vi "Convert_Always_Show_Info.vi"(0 "Array":T9[](array[typedef]) {"ERD Number" format="%.0x"}, 1 "Version":T7, 2 "ATC Data":T3, 5 "Raw Data Out":string[](array[string]), 7 "Previous ERD Info":T8, 9 "ERD Graph Cntrl":T4 {"ERD 1"."Scaler" min=1; "ERD 1"."ERD #" format="%.0x"; "ERD 2"."Scaler" min=1; "ERD 2"."ERD #" format="%.0x"; "ERD 3"."Scaler" min=1; "ERD 3"."ERD #" format="%.0x"}, 11 "Error In":errorcluster) -> (3 "Version":T7, 4 "ERD_Always Show":T8, 6 "Redundant Micro":T6, 8 "ATC Data":T3, 10 "ERD Graph  Ind":T1, 13 "Numeric":i32, 14 "Algorithm Data 2":T2, 15 "Error Out":errorcluster)   [LabVIEW 2014]
doc: "This VI parses the data from ERDs in correct format, units, etc. It handles all hex to dec conversions, hex to enum, and hex to boolean conversions.\n\nIf Raw Data from ERD is blank string, then it will output values from shift register."
uses:
  Utility/LabVIEW GEA2 Toolkit v1.0.0.0/type defs/ERD Read Data Out.ctl
  Utility/LabVIEW GEA2 Toolkit v1.0.0.0/library/GEA2_Toolkit.lvlib
  type defs/ERD_Always_Show.ctl
  type defs/Version.ctl
  type defs/Redundant.ctl
  type defs/ERD_Graph.ctl
  type defs/ERD_Graph_All.ctl
  type defs/ATC_Data.ctl
  type defs/Algorithms.ctl
panel:
  in  "ERD Graph  Ind":T1
  in  "Algorithm Data":T2
  in  "Redundant Micro":T6
  # "Wet Load Size"
  # "Dry Load Size"
  # "OOB"
  # "Wet Load Size"
  # "Dry Load Size"
  # "OOB"
  # "Software Version"
  # "Critical Version"
  # "Non-Critical"
  # "XML Crit Ver"
  # "XML Non-Crit"
  # "Daily Build"
  # "Software Version"
  # "Critical Version"
  # "Non-Critical"
  # "XML Crit Ver"
  # "XML Non-Crit"
  # "Daily Build"
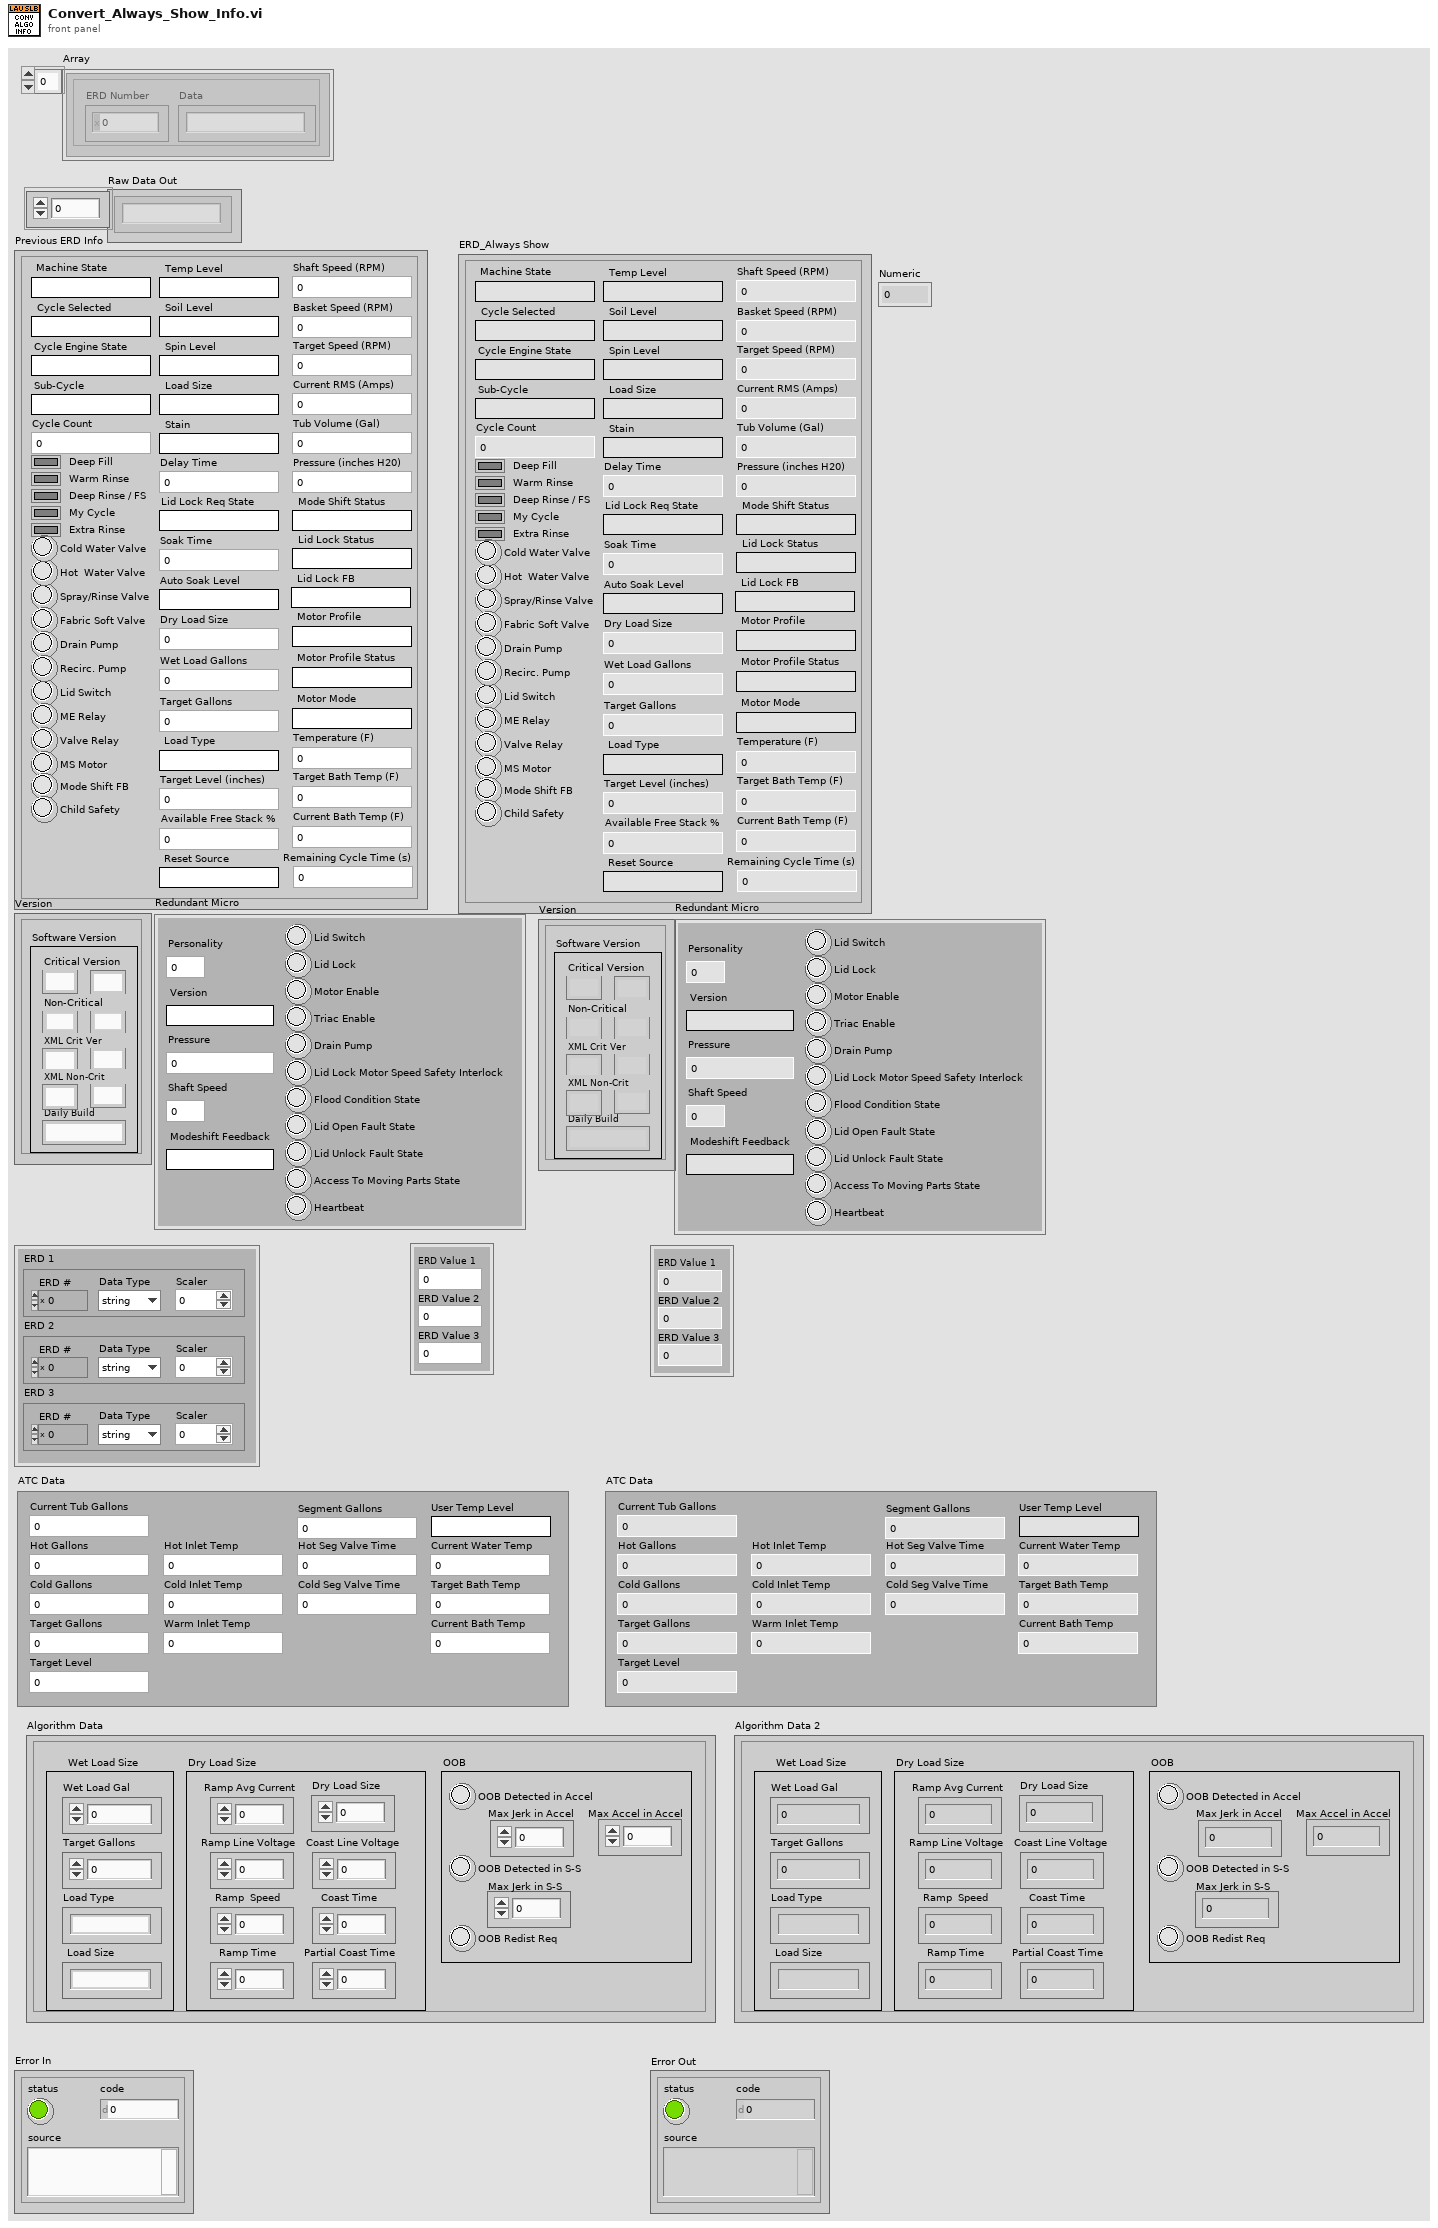
[diagram p1: front panel]
types:
  T1 = cluster{"ERD Value 1":dbl, "ERD Value 2":dbl, "ERD Value 3":dbl}
  T2 = typedef "Algorithms.ctl" = cluster{"Wet Load Gal":dbl, "Target Gallons":dbl, "Load Type":string, "Load Size":string, "Coast Time":u16, "Ramp Time":u16, "Ramp  Speed":u16, "Ramp Avg Current":dbl, "OOB Redist Req":bool, "OOB Detected in S-S":bool, "Max Accel in Accel":i32, "Max Jerk in Accel":i32, "Max Jerk in S-S":i32, "OOB Detected in Accel":bool, "Partial Coast Time":u16, "Dry Load Size":dbl, "Ramp Line Voltage ":dbl, "Coast Line Voltage":dbl}
  T3 = typedef "ATC_Data.ctl" = cluster{"Current Tub Gallons":dbl, "Hot Gallons":dbl, "Cold Gallons":dbl, "Target Gallons":dbl, "Current Water Temp":dbl, "Target Level":u32, "Target Bath Temp":dbl, "Current Bath Temp ":dbl, "Cold Inlet Temp":dbl, "Hot Inlet Temp":dbl, "Warm Inlet Temp":dbl, "Hot Seg Valve Time":u16, "Cold Seg Valve Time ":u16, "User Temp Level":string, "Segment Gallons":dbl}
  T4 = typedef "ERD_Graph_All.ctl" = cluster{"ERD 3":T5, "ERD 2":T5, "ERD 1":T5}
  T5 = typedef "ERD_Graph.ctl" = cluster{"ERD #":u16, "Scaler":u32, "Data Type":enum16{"string", "boolean", "uint8_t", "uint16_t", "uint32_t"}}
  T6 = typedef "Redundant.ctl" = cluster{"Version":string, "Personality":u8, "Pressure ":dbl, "Shaft Speed":u16, "Modeshift Feedback":string, "Lid Switch":bool, "Lid Lock":bool, "Triac Enable":bool, "Drain Pump":bool, "Lid Lock Motor Speed Safety Interlock":bool, "Flood Condition State":bool, "Lid Open Fault State":bool, "Access To Moving Parts State":bool, "Heartbeat":bool, "Motor Enable":bool, "Lid Unlock Fault State":bool}
  T7 = typedef "Version.ctl" = cluster{"Critical Major":string, "Critical Minor":string, "Non-Critical Minor":string, "Non-Critical Major":string, "XML Crit Minor":string, "XMLCrit Major":string, "Daily Rev":string, "XML Non-crit Minor":string, "Xml Non-crit Major":string}
  T8 = typedef "ERD_Always_Show.ctl" = cluster{"Basket Speed (RPM)":u16, "Machine State":string, "Tub Volume (Gal)":dbl, "Pressure (inches H20)":dbl, "Lid Switch ":bool, "Current RMS (Amps)":dbl, "Cycle Selected":string, "Lid Lock Status":string, "Mode Shift Status":string, "Spray/Rinse Valve":bool, "Fabric Soft Valve":bool, "Drain Pump":bool, "Recirc. Pump":bool, "Cycle Engine State":string, "Hot  Water Valve":bool, "Cold Water Valve":bool, "Motor Profile":string, "Motor Profile Status":string, "Motor Mode":string, "ME Relay":bool, "Cycle Count":u32, "Deep Rinse / FS":bool, "My Cycle":bool, "Soil Level":string, "Spin Level":string, "Stain":string, "Temp Level":string, "Load Size":string, "Delay Time":u16, "Soak Time":u16, "Deep Fill":bool, "Warm Rinse":bool, "Auto Soak Level":string, "Extra Rinse":bool, "Wet Load Gallons":dbl, "Target Gallons":dbl, "Sub-Cycle":string, "Load Type":string, "Target Level (inches)":u32, "Valve Relay":bool, "Dry Load Size":dbl, "Shaft Speed (RPM) ":u16, "MS Motor":bool, "Mode Shift FB":bool, "Target Bath Temp (F)":dbl, "Temperature (F)":dbl, "Current Bath Temp (F)":dbl, "Lid Lock FB":string, "Lid Lock Req State":string, "Remaining Cycle Time (s)":dbl, "Available Free Stack %":u8, "Child Safety":bool, "Target Speed (RPM)":u16, "Reset Source":string}
  T9 = typedef "GEA2_Toolkit.lvlib/ERD Read Data Out.ctl" = cluster{"ERD Number":u16, "Data":string}
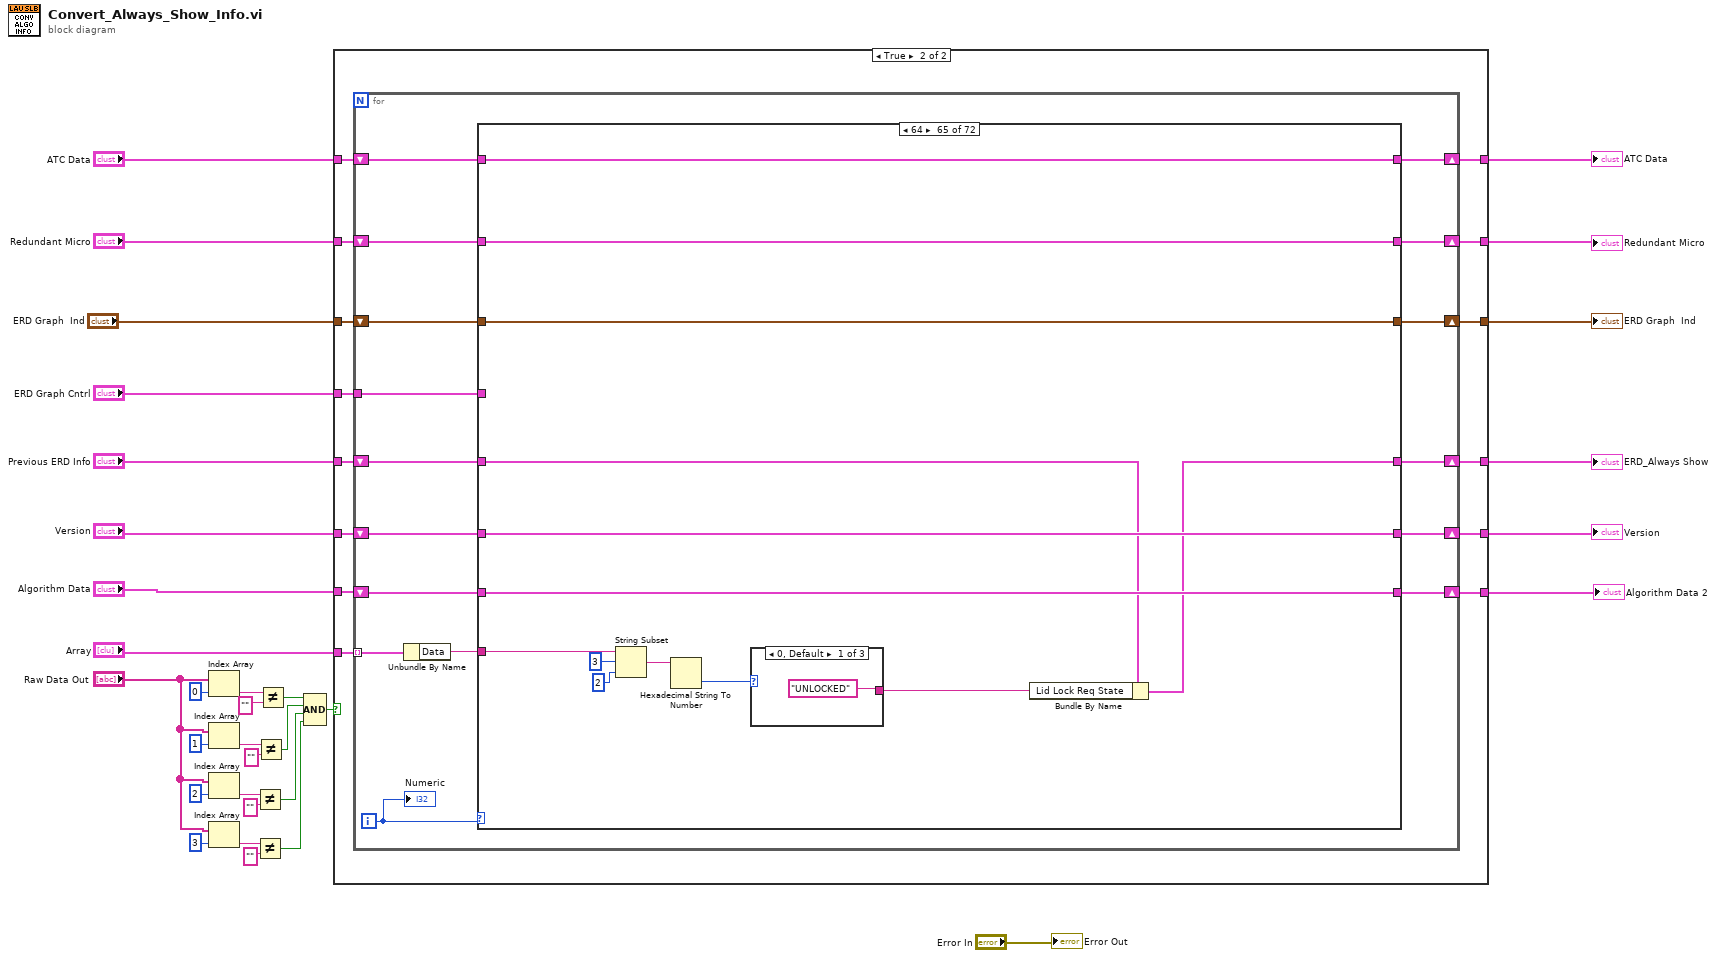
[diagram p0: block diagram]
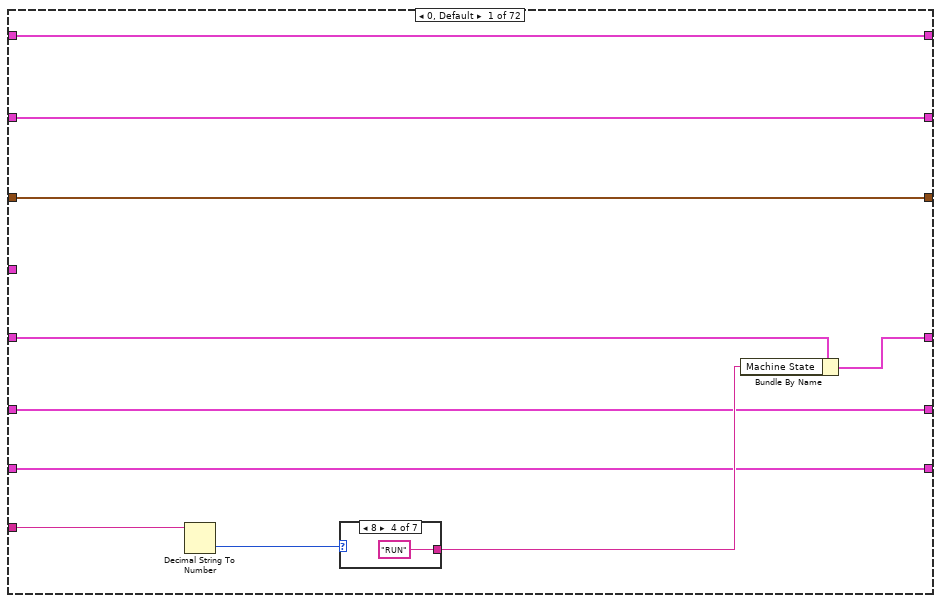
[diagram p3: hidden frame]
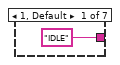
[diagram p4: hidden frame]
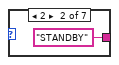
[diagram p5: hidden frame]
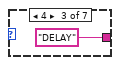
[diagram p6: hidden frame]
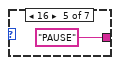
[diagram p7: hidden frame]
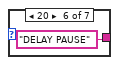
[diagram p8: hidden frame]
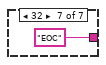
[diagram p9: hidden frame]
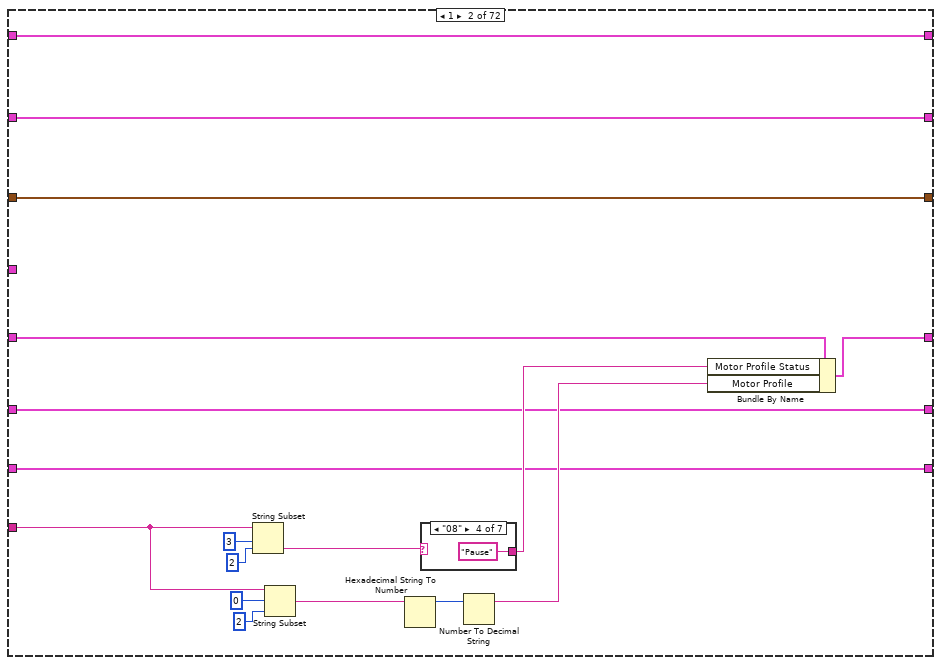
[diagram p10: hidden frame]
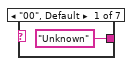
[diagram p11: hidden frame]
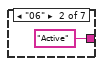
[diagram p12: hidden frame]
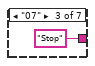
[diagram p13: hidden frame]
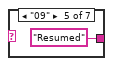
[diagram p14: hidden frame]
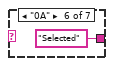
[diagram p15: hidden frame]
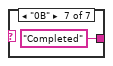
[diagram p16: hidden frame]
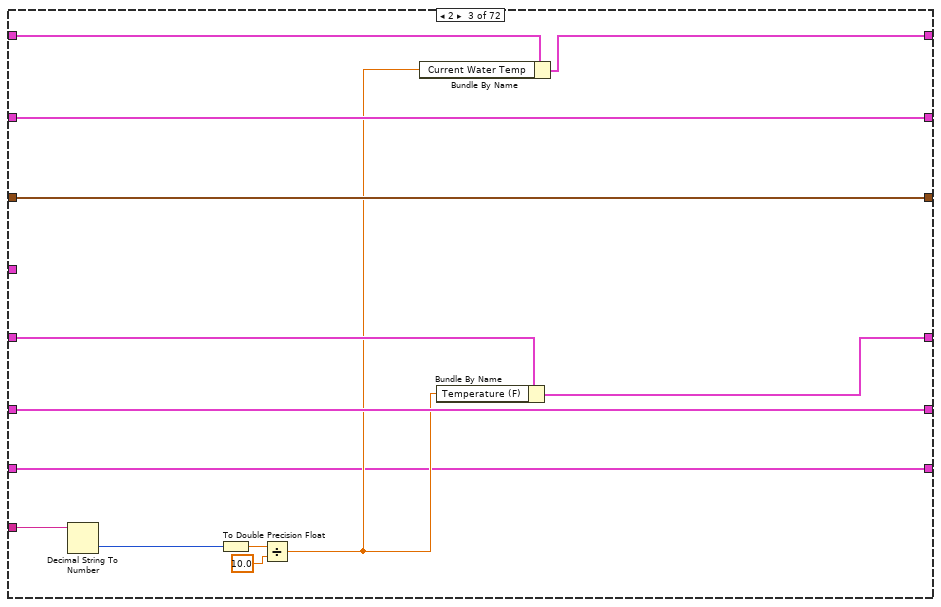
[diagram p17: hidden frame]
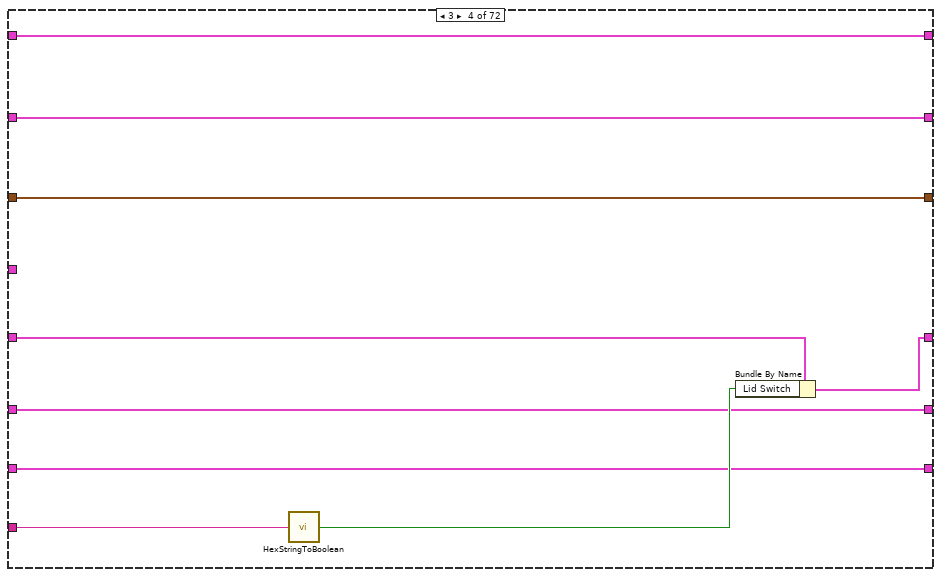
[diagram p18: hidden frame]
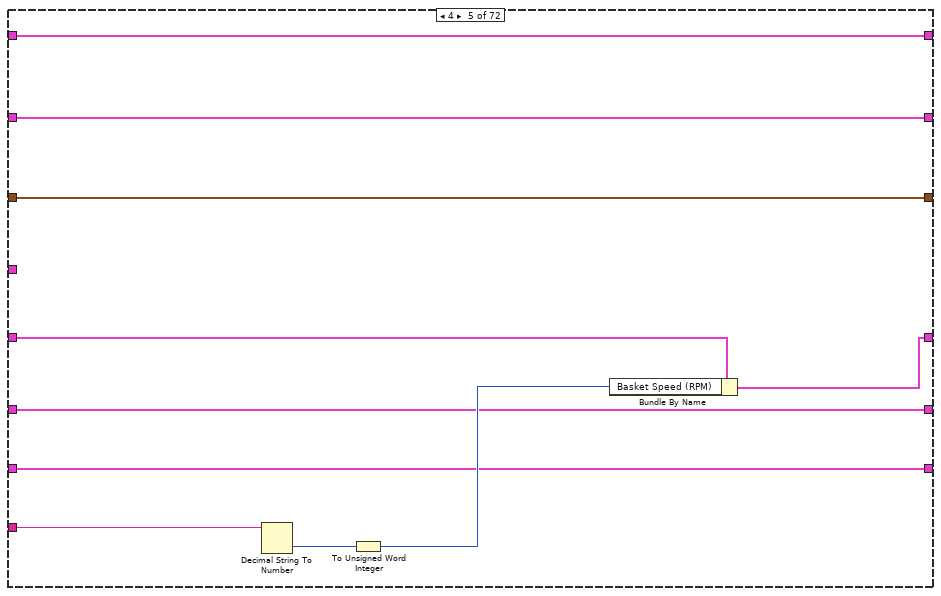
[diagram p19: hidden frame]
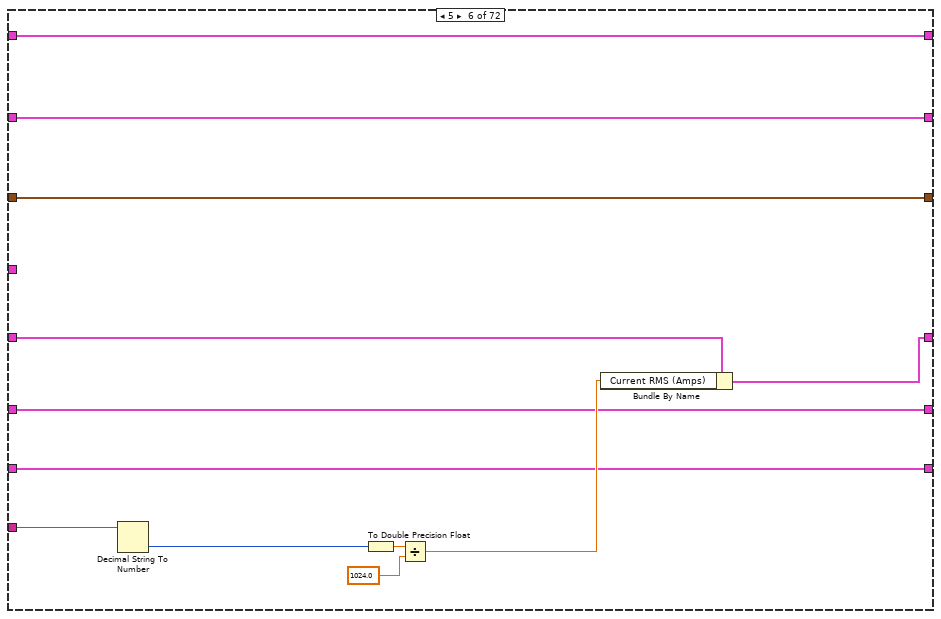
[diagram p20: hidden frame]
diagram:
  n1 = Index Array(array="Raw Data Out", index=0) -> (element=w5:string)
  n2 = Index Array(array="Raw Data Out", index=1) -> (element=w4:string)
  n3 = Index Array(array="Raw Data Out", index=2) -> (element=w2:string)
  n4 = Index Array(array="Raw Data Out", index=3) -> (element=w3:string)
  n5 = Not Equal?(x=w2, y="") -> (x != y?=w8:bool)
  n6 = Not Equal?(x=w3, y="") -> (x != y?=w7:bool)
  n7 = Not Equal?(x=w4, y="") -> (x != y?=w11:bool)
  n8 = Not Equal?(x=w5, y="") -> (x != y?=w16:bool)
  n9 = Compound Arithmetic op=AND(w16, w11, w8, w7) -> (w6:bool)
  n10 = case shown="True" w6 {
    tunnel: "Array" -> [_ w53]
    tunnel: [w34 w52] -> w32
    tunnel: "ERD Graph Cntrl" -> [_ w51]
    tunnel: "Version" -> [w37 w50]
    tunnel: "Previous ERD Info" -> [w38 w49]
    tunnel: [w39 w48] -> w28
    tunnel: [w38 w47] -> w27
    tunnel: [w37 w46] -> w26
    tunnel: "Redundant Micro" -> [w39 w45]
    tunnel: "ATC Data" -> [w36 w44]
    tunnel: [w36 w43] -> w22
    tunnel: "Algorithm Data" -> [w35 w42]
    tunnel: [w35 w41] -> w20
    tunnel: "ERD Graph  Ind" -> [w34 w40]
    frame False {
    }
    frame True {
      n11 = for {
        tunnel: w53 -> [w68] mode=indexing
        shift-right: [w66] -> w47
        shift-left: w49 -> [w65]
        shift-right: [w63] -> w46
        shift-left: w50 -> [w64]
        shift-right: [w61] -> w48
        shift-left: w45 -> [w62]
        shift-right: [w59] -> w52
        shift-left: w40 -> [w58]
        tunnel: w51 -> [w60]
        shift-right: [w56] -> w43
        shift-left: w44 -> [w57]
        shift-right: [w54] -> w41
        shift-left: w42 -> [w55]
        i -> [w69]
        n12 = Unbundle By Name(w68) -> ("Data"=w67:string)
        n13 = case shown="64" w69 {
          tunnel: w67 -> [w76 w94 w120 w131 w141 w150 w164 w176 w185 w214 w225 w239 w256 w268 w279 w306 w323 w341 w351 w358 w367 w382 w388 w400 w408 w417 w424 w435 w451 w466 w482 w495 w515 w525 w532 w543 w556 w571 w583 w606 w619 w632 w658 w678 w688 w701 w714 w726 w740 w754 w768 w775 w804 w816 w828 w844 w865 w875 w885 w896 w907 w917 w929 w941 w961 w976 w978 w1001 w1031 w1033 w1063 w1068]
          tunnel: [w79 w103 w118 w129 w135 w153 w162 w173 w188 w212 w227 w244 w254 w266 w291 w308 w322 w339 w349 w360 w369 w379 w390 w398 w406 w415 w426 w436 w452 w467 w481 w497 w513 w523 w533 w541 w554 w568 w581 w604 w617 w622 w650 w676 w687 w699 w712 w722 w736 w750 w766 w799 w809 w821 w833 w861 w871 w878 w888 w900 w910 w922 w934 w946 w955 w974 w998 w1021 w1029 w1053 w1061 w1074] -> w66
          tunnel: w65 -> [w78 w102 w119 w132 w140 w154 w163 w175 w187 w213 w228 w245 w255 w267 w292 w309 w325 w340 w350 w361 w370 w381 w391 w399 w407 w418 w427 w437 w453 w468 w483 w498 w514 w524 w534 w542 w555 w569 w582 w605 w618 w622 w650 w676 w687 w700 w713 w722 w736 w750 w767 w799 w809 w821 w833 w861 w871 w878 w888 w900 w910 w922 w934 w946 w957 w974 w998 w1021 w1029 w1053 w1061 w1075]
          tunnel: w64 -> [w72 w89 w115 w128 w136 w145 w159 w170 w182 w208 w221 w236 w250 w262 w274 w302 w319 w335 w345 w355 w364 w376 w385 w394 w403 w412 w421 w432 w447 w462 w478 w492 w509 w519 w529 w537 w551 w565 w578 w601 w613 w631 w659 w675 w684 w696 w709 w721 w735 w749 w762 w798 w808 w820 w832 w860 w870 w877 w887 w899 w909 w921 w933 w945 w958 w975 w999 w1022 w1030 w1054 w1062 w1073]
          tunnel: [w72 w89 w115 w128 w136 w145 w159 w170 w182 w208 w221 w236 w250 w262 w274 w302 w319 w335 w345 w355 w364 w376 w385 w394 w403 w412 w421 w432 w447 w462 w478 w492 w509 w519 w529 w537 w551 w565 w578 w601 w613 w625 w653 w675 w684 w696 w709 w721 w735 w749 w762 w798 w808 w820 w832 w860 w870 w877 w887 w899 w909 w921 w933 w945 w958 w975 w999 w1022 w1030 w1054 w1062 w1073] -> w63
          tunnel: w62 -> [w74 w91 w117 w126 w138 w147 w161 w172 w184 w210 w223 w238 w252 w264 w276 w304 w321 w337 w347 w357 w366 w378 w387 w396 w405 w414 w423 w434 w449 w464 w480 w494 w511 w521 w531 w539 w553 w567 w580 w603 w615 w624 w652 w679 w686 w698 w711 w723 w737 w751 w764 w801 w813 w825 w837 w863 w872 w880 w890 w902 w912 w924 w936 w948 w953 w972 w996 w1019 w1027 w1051 w1059 w1065]
          tunnel: [w74 w91 w117 w126 w138 w147 w161 w172 w184 w210 w223 w238 w252 w264 w276 w304 w321 w337 w347 w357 w366 w378 w387 w396 w405 w414 w423 w434 w449 w464 w480 w494 w511 w521 w531 w539 w553 w567 w580 w603 w615 w624 w652 w677 w686 w698 w711 w723 w737 w751 w764 w801 w813 w825 w837 w863 w872 w880 w890 w902 w912 w924 w936 w948 w953 w972 w996 w1019 w1027 w1051 w1059 w1065] -> w61
          tunnel: w60 -> [_ _ _ _ _ _ _ _ _ _ _ _ _ _ _ _ _ _ _ _ _ _ _ _ _ _ _ _ _ _ _ _ _ _ _ _ _ _ _ _ _ _ _ _ _ _ _ w728 w742 w756 _ _ _ _ _ _ _ _ _ _ _ _ _ _ _ _ _ _ _ _ _ _]
          tunnel: [w73 w90 w116 w127 w137 w146 w160 w171 w183 w209 w222 w237 w251 w263 w275 w303 w320 w336 w346 w356 w365 w377 w386 w395 w404 w413 w422 w433 w448 w463 w479 w493 w510 w520 w530 w538 w552 w566 w579 w602 w614 w623 w651 w674 w685 w697 w710 w724 w738 w752 w763 w800 w810 w822 w834 w862 w867 w879 w889 w901 w911 w923 w935 w947 w954 w973 w997 w1020 w1028 w1052 w1060 w1066] -> w59
          tunnel: w58 -> [w73 w90 w116 w127 w137 w146 w160 w171 w183 w209 w222 w237 w251 w263 w275 w303 w320 w336 w346 w356 w365 w377 w386 w395 w404 w413 w422 w433 w448 w463 w479 w493 w510 w520 w530 w538 w552 w566 w579 w602 w614 w623 w651 w674 w685 w697 w710 w718 w732 w746 w763 w800 w810 w822 w834 w862 w867 w879 w889 w901 w911 w923 w935 w947 w954 w973 w997 w1020 w1028 w1052 w1060 w1066]
          tunnel: w57 -> [w71 w88 w114 w125 w134 w144 w158 w169 w181 w207 w220 w235 w249 w261 w273 w301 w318 w334 w344 w354 w363 w375 w384 w393 w402 w411 w420 w431 w446 w461 w477 w491 w508 w518 w528 w536 w550 w564 w577 w600 w612 w621 w649 w673 w682 w695 w708 w720 w734 w748 w761 w787 w812 w824 w836 w852 w873 w881 w891 w903 w913 w925 w937 w949 w952 w971 w995 w1018 w1026 w1050 w1058 w1064]
          tunnel: [w71 w88 w113 w125 w134 w144 w157 w169 w181 w207 w220 w235 w249 w261 w273 w301 w318 w334 w344 w354 w363 w375 w384 w393 w402 w411 w420 w430 w446 w461 w477 w491 w508 w518 w528 w536 w550 w563 w577 w599 w612 w621 w649 w673 w681 w694 w707 w720 w734 w748 w761 w773 w811 w823 w835 w843 w873 w881 w891 w903 w913 w925 w937 w949 w952 w971 w995 w1018 w1026 w1050 w1058 w1064] -> w56
          tunnel: w55 -> [w70 w87 w111 w124 w133 w143 w155 w168 w180 w206 w219 w234 w248 w260 w272 w300 w317 w333 w343 w353 w362 w374 w383 w392 w401 w410 w419 w428 w445 w460 w476 w490 w507 w517 w527 w535 w549 w562 w576 w597 w611 w620 w648 w672 w683 w692 w705 w719 w733 w747 w760 w772 w802 w814 w826 w838 w869 w883 w893 w905 w915 w927 w939 w951 w959 w970 w994 w1017 w1025 w1049 w1057 w1072]
          tunnel: [w70 w87 w111 w124 w133 w143 w155 w168 w180 w206 w219 w234 w248 w260 w272 w300 w317 w333 w343 w353 w362 w374 w383 w392 w401 w410 w419 w428 w445 w460 w475 w490 w507 w517 w527 w535 w548 w561 w575 w597 w611 w620 w648 w672 w683 w692 w705 w719 w733 w747 w760 w772 w802 w814 w826 w838 w868 w882 w892 w904 w914 w926 w938 w950 w959 w969 w993 w1016 w1024 w1048 w1056 w1072] -> w54
          frame 0, Default {
            n14 = Decimal String To Number(string=w76) -> (number=w77:i32)  [unwired: 2 in, 1 out]
            n15 = case shown="8" w77 {
              tunnel: ["IDLE" "STANDBY" "DELAY" "RUN" "PAUSE" "DELAY PAUSE" ("Profile Status") "EOC"] -> w75
              frame 1, Default {
              }
              frame 2 {
              }
              frame 4 {
              }
              frame 8 {
              }
              frame 16 {
              }
              frame 20 {
              }
              frame 32 {
              }
            }
            n16 = Bundle By Name(cluster=w78, "Machine State"=w75) -> (w79:T8)
          }
          frame 1 {
            n17 = String Subset(string=w94, offset (0)=3, length (rest)=2 ("length (rest)")) -> (substring=w99:string)
            n18 = String Subset(string=w94, offset (0)=0, length (rest)=2 ("length (rest)")) -> (substring=w96:string)
            n19 = Hexadecimal String To Number(string=w96) -> (number=w95:u32)  [unwired: 2 in, 1 out]
            n20 = case shown="\"08\"" w99 {
              tunnel: ["Unknown" ("Profile Status") "Active" ("Profile Status") "Stop" ("Profile Status") "Pause" ("Profile Status") "Resumed" ("Profile Status") "Selected" ("Profile Status") "Completed" ("Profile Status")] -> w93
              frame "00", Default {
              }
              frame "06" {
              }
              frame "07" {
              }
              frame "08" {
              }
              frame "09" {
              }
              frame "0A" {
              }
              frame "0B" {
              }
            }
            n21 = Number To Decimal String(number=w95) -> (decimal integer string=w92:string)  [unwired: 1 in]
            n22 = Bundle By Name(cluster=w102, "Motor Profile Status"=w93, "Motor Profile"=w92) -> (w103:T8)
          }
          frame 2 {
            n23 = Decimal String To Number(string=w120) -> (number=w121:i32)  [unwired: 2 in, 1 out]
            n24 = To Double Precision Float(number=w121) -> (double precision float=w123:dbl)
            n25 = Divide(x=w123, y=10.0) -> (x/y=w112:dbl)
            n26 = Bundle By Name(cluster=w114, "Current Water Temp"=w112) -> (w113:T3)
            n27 = Bundle By Name(cluster=w119, "Temperature (F)"=w112) -> (w118:T8)
          }
          frame 3 {
            n28 = call "HexStringToBoolean.vi"("Hex String"=w131) -> ("Boolean"=w130:bool)
            n29 = Bundle By Name(cluster=w132, "Lid Switch"=w130) -> (w129:T8)
          }
          frame 4 {
            n30 = Decimal String To Number(string=w141) -> (number=w142:i32)  [unwired: 2 in, 1 out]
            n31 = To Unsigned Word Integer(number=w142) -> (unsigned 16bit integer=w139:u16)
            n32 = Bundle By Name(cluster=w140, "Basket Speed (RPM)"=w139) -> (w135:T8)
          }
          frame 5 {
            n33 = Decimal String To Number(string=w150) -> (number=w151:i32)  [unwired: 2 in, 1 out]
            n34 = To Double Precision Float(number=w151) -> (double precision float=w152:dbl)
            n35 = Divide(x=w152, y=1024.0) -> (x/y=w148:dbl)
            n36 = Bundle By Name(cluster=w154, "Current RMS (Amps)"=w148) -> (w153:T8)
          }
          frame 6 {
            n37 = Decimal String To Number(string=w164) -> (number=w165:i32)  [unwired: 2 in, 1 out]
            n38 = To Double Precision Float(number=w165) -> (double precision float=w166:dbl)
            n39 = Divide(x=w166, y=100.0) -> (x/y=w156:dbl)
            n40 = Bundle By Name(cluster=w158, "Current Tub Gallons"=w156) -> (w157:T3)
            n41 = Bundle By Name(cluster=w163, "Tub Volume (Gal)"=w156) -> (w162:T8)
          }
          frame 7 {
            n42 = Decimal String To Number(string=w176) -> (number=w177:i32)  [unwired: 2 in, 1 out]
            n43 = To Double Precision Float(number=w177) -> (double precision float=w179:dbl)
            n44 = Divide(x=w179, y=1000.0) -> (x/y=w174:dbl)
            n45 = Bundle By Name(cluster=w175, "Pressure (inches H20)"=w174) -> (w173:T8)
          }
          frame 8 {
            n46 = Decimal String To Number(string=w185) -> (number=w189:i32)  [unwired: 2 in, 1 out]
            n47 = case shown="2" w189 {
              tunnel: ["Cycle 0" ("Motor Profile") "Cycle 1" ("Motor Profile") "Cycle 2" ("Motor Profile") "Cycle 3" ("Motor Profile") "Cycle 4" ("Motor Profile") "Cycle 5" ("Motor Profile") "Cycle 6" ("Motor Profile") "Cycle 7" ("Motor Profile") "Cycle 8" ("Motor Profile") "Cycle 9" ("Motor Profile") "Cycle 10" ("Motor Profile") "Cycle 11" ("Motor Profile") "Cycle 12" ("Motor Profile") "Cycle 13" ("Motor Profile") "Cycle 14" ("Motor Profile") "Cycle 15" ("Motor Profile")] -> w186
              frame 0, Default {
              }
              frame 1 {
              }
              frame 2 {
              }
              frame 3 {
              }
              frame 4 {
              }
              frame 5 {
              }
              frame 6 {
              }
              frame 7 {
              }
              frame 8 {
              }
              frame 9 {
              }
              frame 10 {
              }
              frame 11 {
              }
              frame 12 {
              }
              frame 13 {
              }
              frame 14 {
              }
              frame 15 {
              }
            }
            n48 = Bundle By Name(cluster=w187, "Cycle Selected"=w186) -> (w188:T8)
          }
          frame 9 {
            n49 = Decimal String To Number(string=w214) -> (number=w215:i32)  [unwired: 2 in, 1 out]
            n50 = case shown="2" w215 {
              tunnel: ["Unlocked" ("Motor Profile") "Locked" ("Motor Profile") "Failure" ("Motor Profile")] -> w211
              frame 0, Default {
              }
              frame 1 {
              }
              frame 2 {
              }
            }
            n51 = Bundle By Name(cluster=w213, "Lid Lock Status"=w211) -> (w212:T8)
          }
          frame 10 {
            n52 = Decimal String To Number(string=w225) -> (number=w226:i32)  [unwired: 2 in, 1 out]
            n53 = case shown="4" w226 {
              tunnel: ["Unknown" ("Motor Profile") "Agitate State" ("Motor Profile") "Spin State" ("Motor Profile") "Trans to Spin" ("Motor Profile") "Trans to Agitate" ("Motor Profile")] -> w224
              frame 0, Default {
              }
              frame 1 {
              }
              frame 2 {
              }
              frame 3 {
              }
              frame 4 {
              }
            }
            n54 = Bundle By Name(cluster=w228, "Mode Shift Status"=w224) -> (w227:T8)
          }
          frame 11 {
            n55 = Decimal String To Number(string=w239) -> (number=w246:i32)  [unwired: 2 in, 1 out]
            n56 = Number To Boolean Array(number=w246) -> (Boolean array=w247:bool[])
            n57 = Index Array(array=w247) -> (element #1=w243:bool, element #2=w242:bool, element #3=w241:bool, element #4=w240:bool)  [unwired: 4 in]
            n58 = Bundle By Name(cluster=w245, "Hot  Water Valve"=w243, "Cold Water Valve"=w242, "Spray/Rinse Valve"=w241, "Fabric Soft Valve"=w240) -> (w244:T8)
          }
          frame 12 {
            n59 = String Subset(string=w256, offset (0)=3, length (rest)=2 ("length (rest)")) -> (substring=w257:string)
            n60 = call "HexStringToBoolean.vi"("Hex String"=w257) -> ("Boolean"=w253:bool)
            n61 = Bundle By Name(cluster=w255, "Drain Pump"=w253) -> (w254:T8)
          }
          frame 13 {
            n62 = String Subset(string=w268, offset (0)=3, length (rest)=2 ("length (rest)")) -> (substring=w269:string)
            n63 = call "HexStringToBoolean.vi"("Hex String"=w269) -> ("Boolean"=w265:bool)
            n64 = Bundle By Name(cluster=w267, "Recirc. Pump"=w265) -> (w266:T8)
          }
          frame 14 {
            n65 = String Subset(string=w279, offset (0)=3, length (rest)=2 ("length (rest)")) -> (substring=w283:string)
            n66 = String Subset(string=w279, offset (0)=0, length (rest)=2 ("length (rest)")) -> (substring=w286:string)
            n67 = Hexadecimal String To Number(string=w286) -> (number=w285:u32)  [unwired: 2 in, 1 out]
            n68 = Hexadecimal String To Number(string=w283) -> (number=w281:u32)  [unwired: 2 in, 1 out]
            n69 = case shown="0, Default" w281 {
              tunnel: ["Unknown" "Started" "Stopped" "Paused" "Resumed" "Selected" "Completed"] -> w282
              frame 0, Default {
              }
              frame 6 {
              }
              frame 7 {
              }
              frame 8 {
              }
              frame 9 {
              }
              frame 10 {
              }
              frame 11 {
              }
            }
            n70 = Number To Decimal String(number=w285) -> (decimal integer string=w284:string)  [unwired: 1 in]
            n71 = call <vilib>:"Space Constant.vi"() -> ("String"=w280:string)
            n72 = Concatenate Strings("Cycle" ("string"), w280, w284, w280, w282) -> (w277:string)
            n73 = Bundle By Name(cluster=w292, "Cycle Engine State"=w277) -> (w291:T8)
          }
          frame 15 {
            n74 = Decimal String To Number(string=w306) -> (number=w307:i32)  [unwired: 2 in, 1 out]
            n75 = case shown="0, Default" w307 {
              tunnel: ["Closed Loop" "Closed Loop Angle" "Open Loop" "Open Loop Angle" "Coasting" "Braking" "Idle"] -> w305
              frame 0, Default {
              }
              frame 1 {
              }
              frame 2 {
              }
              frame 3 {
              }
              frame 4 {
              }
              frame 5 {
              }
              frame 6 {
              }
            }
            n76 = Bundle By Name(cluster=w309, "Motor Mode"=w305) -> (w308:T8)
          }
          frame 16 {
            n77 = case shown="\"00\"" w323 {
              selector: w323 -> [w326 _ _ _ _ _ _]
              tunnel: [w326 "NONE" "FILL" "SOAK" "WASH" "RINSE" "SPIN"] -> w324
              frame Default {
              }
              frame "00" {
              }
              frame "01" {
              }
              frame "02" {
              }
              frame "04" {
              }
              frame "08" {
              }
              frame "10" {
              }
            }
            n78 = Bundle By Name(cluster=w325, "Sub-Cycle"=w324) -> (w322:T8)
          }
          frame 17 {
            n79 = Decimal String To Number(string=w341) -> (number=w342:i32)  [unwired: 2 in, 1 out]
            n80 = To Unsigned Long Integer(number=w342) -> (unsigned 32bit integer=w338:u32)
            n81 = Bundle By Name(cluster=w340, "Cycle Count"=w338) -> (w339:T8)
          }
          frame 18 {
            n82 = Decimal String To Number(string=w351) -> (number=w352:i32)  [unwired: 2 in, 1 out]
            n83 = To Unsigned Word Integer(number=w352) -> (unsigned 16bit integer=w348:u16)
            n84 = Bundle By Name(cluster=w350, "Shaft Speed (RPM)"=w348) -> (w349:T8)
          }
          frame 19 {
            n85 = call "HexStringToBoolean.vi"("Hex String"=w358) -> ("Boolean"=w359:bool)
            n86 = Bundle By Name(cluster=w361, "ME Relay"=w359) -> (w360:T8)
          }
          frame 20 {
            n87 = String Subset(string=w367, offset (0)=3, length (rest)=2 ("length (rest)")) -> (substring=w371:string)
            n88 = call "HexStringToBoolean.vi"("Hex String"=w371) -> ("Boolean"=w368:bool)
            n89 = Bundle By Name(cluster=w370, "Valve Relay"=w368) -> (w369:T8)
          }
          frame 21 {
            n90 = call "HexStringToBoolean.vi"("Hex String"=w382) -> ("Boolean"=w380:bool)
            n91 = Bundle By Name(cluster=w381, "MS Motor"=w380) -> (w379:T8)
          }
          frame 22 {
            n92 = call "HexStringToBoolean.vi"("Hex String"=w388) -> ("Boolean"=w389:bool)
            n93 = Bundle By Name(cluster=w391, "Deep Fill"=w389) -> (w390:T8)
          }
          frame 23 {
            n94 = call "HexStringToBoolean.vi"("Hex String"=w400) -> ("Boolean"=w397:bool)
            n95 = Bundle By Name(cluster=w399, "Warm Rinse"=w397) -> (w398:T8)
          }
          frame 24 {
            n96 = call "HexStringToBoolean.vi"("Hex String"=w408) -> ("Boolean"=w409:bool)
            n97 = Bundle By Name(cluster=w407, "Deep Rinse / FS"=w409) -> (w406:T8)
          }
          frame 25 {
            n98 = call "HexStringToBoolean.vi"("Hex String"=w417) -> ("Boolean"=w416:bool)
            n99 = Bundle By Name(cluster=w418, "My Cycle"=w416) -> (w415:T8)
          }
          frame 26 {
            n100 = call "HexStringToBoolean.vi"("Hex String"=w424) -> ("Boolean"=w425:bool)
            n101 = Bundle By Name(cluster=w427, "Extra Rinse"=w425) -> (w426:T8)
          }
          frame 27 {
            n102 = case shown="\"01\"" w435 {
              selector: w435 -> [w438 _ _ _ _ _ _]
              tunnel: [w438 "TAP COLD" "COLD" "COOL" "COLORS" "WARM" "HOT"] -> w429
              frame Default {
              }
              frame "00" {
              }
              frame "01" {
              }
              frame "02" {
              }
              frame "03" {
              }
              frame "04" {
              }
              frame "05" {
              }
            }
            n103 = Bundle By Name(cluster=w431, "User Temp Level"=w429) -> (w430:T3)
            n104 = Bundle By Name(cluster=w437, "Temp Level"=w429) -> (w436:T8)
          }
          frame 28 {
            n105 = case shown="\"00\"" w451 {
              selector: w451 -> [w454 _ _ _ _ _]
              tunnel: [w454 "EXTRA LIGHT" "LIGHT" "NORMAL" "HEAVY" "EXTRA HEAVY"] -> w450
              frame Default {
              }
              frame "00" {
              }
              frame "01" {
              }
              frame "02" {
              }
              frame "03" {
              }
              frame "04" {
              }
            }
            n106 = Bundle By Name(cluster=w453, "Soil Level"=w450) -> (w452:T8)
          }
          frame 29 {
            n107 = case shown="\"03\"" w466 {
              selector: w466 -> [w469 _ _ _ _]
              tunnel: [w469 "NO SPIN" "NORMAL" "MORE " "MAX"] -> w465
              frame Default {
              }
              frame "00" {
              }
              frame "01" {
              }
              frame "02" {
              }
              frame "03" {
              }
            }
            n108 = Bundle By Name(cluster=w468, "Spin Level"=w465) -> (w467:T8)
          }
          frame 30 {
            n109 = case shown="\"04\"" w482 {
              selector: w482 -> [w484 _ _ _ _ _]
              tunnel: [w484 "SMALL" "MEDIUM" "LARGE" "SUPER" "PRECISE FILL"] -> w474
              frame Default {
              }
              frame "00" {
              }
              frame "01" {
              }
              frame "02" {
              }
              frame "03" {
              }
              frame "04" {
              }
            }
            n110 = Bundle By Name(cluster=w476, "Load Size"=w474) -> (w475:T2)
            n111 = Bundle By Name(cluster=w483, "Load Size"=w474) -> (w481:T8)
          }
          frame 31 {
            n112 = case shown="\"01\"" w495 {
              selector: w495 -> [w499 _ _ _ _ _ _ _]
              tunnel: [w499 "OFF" "TOMATO" "WINE" "BLOOD" "OILY" "GRASS" "DIRT"] -> w496
              frame Default {
              }
              frame "00" {
              }
              frame "01" {
              }
              frame "02" {
              }
              frame "03" {
              }
              frame "04" {
              }
              frame "05" {
              }
              frame "06" {
              }
            }
            n113 = Bundle By Name(cluster=w498, "Stain"=w496) -> (w497:T8)
          }
          frame 32 {
            n114 = Decimal String To Number(string=w515) -> (number=w516:i32)  [unwired: 2 in, 1 out]
            n115 = To Unsigned Word Integer(number=w516) -> (unsigned 16bit integer=w512:u16)
            n116 = Bundle By Name(cluster=w514, "Delay Time"=w512) -> (w513:T8)
          }
          frame 33 {
            n117 = Decimal String To Number(string=w525) -> (number=w526:i32)  [unwired: 2 in, 1 out]
            n118 = To Unsigned Word Integer(number=w526) -> (unsigned 16bit integer=w522:u16)
            n119 = Bundle By Name(cluster=w524, "Soak Time"=w522) -> (w523:T8)
          }
          frame 34 {
            n120 = Bundle By Name(cluster=w534, "Auto Soak Level"=w532) -> (w533:T8)
          }
          frame 35 {
            n121 = Decimal String To Number(string=w543) -> (number=w546:i32)  [unwired: 2 in, 1 out]
            n122 = To Double Precision Float(number=w546) -> (double precision float=w545:dbl)
            n123 = Divide(x=w545, y=32.0) -> (x/y=w540:dbl)
            n124 = Bundle By Name(cluster=w542, "Dry Load Size"=w540) -> (w541:T8)
          }
          frame 36 {
            n125 = Decimal String To Number(string=w556) -> (number=w559:i32)  [unwired: 2 in, 1 out]
            n126 = To Double Precision Float(number=w559) -> (double precision float=w558:dbl)
            n127 = Divide(x=w558, y=100.0) -> (x/y=w547:dbl)
            n128 = Bundle By Name(cluster=w549, "Wet Load Gal"=w547) -> (w548:T2)
            n129 = Bundle By Name(cluster=w555, "Wet Load Gallons"=w547) -> (w554:T8)
          }
          frame 37 {
            n130 = Decimal String To Number(string=w571) -> (number=w572:i32)  [unwired: 2 in, 1 out]
            n131 = To Double Precision Float(number=w572) -> (double precision float=w573:dbl)
            n132 = Divide(x=w573, y=100.0) -> (x/y=w560:dbl)
            n133 = Bundle By Name(cluster=w564, "Target Gallons"=w560) -> (w563:T3)
            n134 = Bundle By Name(cluster=w569, "Target Gallons"=w560) -> (w568:T8)
            n135 = Bundle By Name(cluster=w562, "Target Gallons"=w560) -> (w561:T2)
          }
          frame 38 {
            n136 = case shown="\"11\"" w583 {
              selector: w583 -> [w584 _ _ _ _ _ _ _ _ _ _ _ _]
              tunnel: [w584 "UNKNOWN" "COTTON" "SYNTHETIC" "MIXED" "WET" "LOW FLOW" "SMALL" "MEDIUM" "LARGE" "SUPER" "SUPER PLUS" "MAX"] -> w574
              frame Default {
              }
              frame "0" {
              }
              frame "1" {
              }
              frame "2" {
              }
              frame "3" {
              }
              frame "4" {
              }
              frame "5" {
              }
              frame "6" {
              }
              frame "7" {
              }
              frame "8" {
              }
              frame "9" {
              }
              frame "10" {
              }
              frame "11" {
              }
            }
            n137 = Bundle By Name(cluster=w576, "Load Type"=w574) -> (w575:T2)
            n138 = Bundle By Name(cluster=w582, "Load Type"=w574) -> (w581:T8)
          }
          frame 39 {
            n139 = Decimal String To Number(string=w606) -> (number=w610:i32)  [unwired: 2 in, 1 out]
            n140 = To Double Precision Float(number=w610) -> (double precision float=w608:dbl)
            n141 = Divide(x=w608, y=1000.0) -> (x/y=w609:dbl)
            n142 = To Unsigned Long Integer(number=w609) -> (unsigned 32bit integer=w598:u32)
            n143 = Bundle By Name(cluster=w600, "Target Level"=w598) -> (w599:T3)
            n144 = Bundle By Name(cluster=w605, "Target Level (inches)"=w598) -> (w604:T8)
          }
          frame 40 {
            n145 = call "HexStringToBoolean.vi"("Hex String"=w619) -> ("Boolean"=w616:bool)
            n146 = Bundle By Name(cluster=w618, "Mode Shift FB"=w616) -> (w617:T8)
          }
          frame 41 {
            w633 = 2 ("length (rest)")
            n147 = String Subset(string=w632, offset (0)=0 ("length (rest)"), length (rest)=w633) -> (substring=w647:string)
            n148 = String Subset(string=w632, offset (0)=3 ("length (rest)"), length (rest)=w633) -> (substring=w643:string)
            n149 = String Subset(string=w632, offset (0)=6 ("length (rest)"), length (rest)=w633) -> (substring=w638:string)
            n150 = String Subset(string=w632, offset (0)=9 ("length (rest)"), length (rest)=w633) -> (substring=w637:string)
            n151 = Hexadecimal String To Number(string=w647) -> (number=w642:u32)  [unwired: 2 in, 1 out]
            n152 = Hexadecimal String To Number(string=w643) -> (number=w641:u32)  [unwired: 2 in, 1 out]
            n153 = Hexadecimal String To Number(string=w638) -> (number=w640:u32)  [unwired: 2 in, 1 out]
            n154 = Hexadecimal String To Number(string=w637) -> (number=w639:u32)  [unwired: 2 in, 1 out]
            n155 = Concatenate Strings(w638, w637) -> (w636:string)
            n156 = Number To Decimal String(number=w642) -> (decimal integer string=w630:string)  [unwired: 1 in]
            n157 = Number To Decimal String(number=w641) -> (decimal integer string=w629:string)  [unwired: 1 in]
            n158 = Number To Decimal String(number=w640) -> (decimal integer string=w628:string)  [unwired: 1 in]
            n159 = Number To Decimal String(number=w639) -> (decimal integer string=w627:string)  [unwired: 1 in]
            n160 = Hexadecimal String To Number(string=w636) -> (number=w635:u32)  [unwired: 2 in, 1 out]
            n161 = Number To Decimal String(number=w635) -> (decimal integer string=w626:string)  [unwired: 1 in]
            n162 = Bundle By Name(cluster=w631, "Critical Major"=w630, "Critical Minor"=w629, "Non-Critical Major"=w628, "Non-Critical Minor"=w627, "Daily Rev"=w626) -> (w625:T7)
          }
          frame 42 {
            n163 = String Subset(string=w658, offset (0)=0 ("length (rest)")) -> (substring=w669:string)  [unwired: 1 in]
            n164 = String Subset(string=w658, offset (0)=3 ("length (rest)")) -> (substring=w668:string)  [unwired: 1 in]
            n165 = String Subset(string=w658, offset (0)=6) -> (substring=w665:string)  [unwired: 1 in]
            n166 = String Subset(string=w658, offset (0)=9) -> (substring=w664:string)  [unwired: 1 in]
            n167 = Hexadecimal String To Number(string=w669) -> (number=w667:u32)  [unwired: 2 in, 1 out]
            n168 = Hexadecimal String To Number(string=w668) -> (number=w666:u32)  [unwired: 2 in, 1 out]
            n169 = Hexadecimal String To Number(string=w665) -> (number=w663:u32)  [unwired: 2 in, 1 out]
            n170 = Hexadecimal String To Number(string=w664) -> (number=w660:u32)  [unwired: 2 in, 1 out]
            n171 = Number To Decimal String(number=w667) -> (decimal integer string=w657:string)  [unwired: 1 in]
            n172 = Number To Decimal String(number=w666) -> (decimal integer string=w656:string)  [unwired: 1 in]
            n173 = Number To Decimal String(number=w663) -> (decimal integer string=w655:string)  [unwired: 1 in]
            n174 = Number To Decimal String(number=w660) -> (decimal integer string=w654:string)  [unwired: 1 in]
            n175 = Bundle By Name(cluster=w659, "XMLCrit Major"=w657, "XML Crit Minor"=w656, "Xml Non-crit Major"=w655, "XML Non-crit Minor"=w654) -> (w653:T7)
          }
          frame 43 {
            n176 = call "Red_Micro_Parse.vi"("Data"=w678, "Redundant Micro in"=w679) -> ("Redundant Micro out"=w677:T6)  [unwired: 9 in]
          }
          frame 44 {
            n177 = Decimal String To Number(string=w688) -> (number=w689:i32)  [unwired: 2 in, 1 out]
            n178 = To Double Precision Float(number=w689) -> (double precision float=w691:dbl)
            n179 = Divide(x=w691, y=100.0) -> (x/y=w680:dbl)
            n180 = Bundle By Name(cluster=w682, "Segment Gallons"=w680) -> (w681:T3)
          }
          frame 45 {
            (unwired) 10.0 ("y")
            n181 = Decimal String To Number(string=w701) -> (number=w704:i32)  [unwired: 2 in, 1 out]
            n182 = To Double Precision Float(number=w704) -> (double precision float=w702:dbl)
            n183 = Divide(x=w702, y=10.0) -> (x/y=w693:dbl)
            n184 = Bundle By Name(cluster=w695, "Target Bath Temp"=w693) -> (w694:T3)
            n185 = Bundle By Name(cluster=w700, "Target Bath Temp (F)"=w693) -> (w699:T8)
          }
          frame 46 {
            n186 = Decimal String To Number(string=w714) -> (number=w715:i32)  [unwired: 2 in, 1 out]
            n187 = To Double Precision Float(number=w715) -> (double precision float=w717:dbl)
            n188 = Divide(x=w717, y=10.0) -> (x/y=w706:dbl)
            n189 = Bundle By Name(cluster=w708, "Current Bath Temp"=w706) -> (w707:T3)
            n190 = Bundle By Name(cluster=w713, "Current Bath Temp (F)"=w706) -> (w712:T8)
          }
          frame 47 {
            n191 = Unbundle By Name(w728) -> ("ERD 1.Scaler"=w727:u32)
            n192 = Decimal String To Number(string=w726) -> (number=w729:i32)  [unwired: 2 in, 1 out]
            n193 = To Double Precision Float(number=w727) -> (double precision float=w730:dbl)
            n194 = To Double Precision Float(number=w729) -> (double precision float=w731:dbl)
            n195 = Divide(x=w731, y=w730) -> (x/y=w725:dbl)
            n196 = Bundle By Name(cluster=w718, "ERD Value 1"=w725) -> (w724:T1)
          }
          frame 48 {
            n197 = Unbundle By Name(w742) -> ("ERD 2.Scaler"=w741:u32)
            n198 = Decimal String To Number(string=w740) -> (number=w743:i32)  [unwired: 2 in, 1 out]
            n199 = To Double Precision Float(number=w741) -> (double precision float=w744:dbl)
            n200 = To Double Precision Float(number=w743) -> (double precision float=w745:dbl)
            n201 = Divide(x=w745, y=w744) -> (x/y=w739:dbl)
            n202 = Bundle By Name(cluster=w732, "ERD Value 2"=w739) -> (w738:T1)
          }
          frame 49 {
            n203 = Unbundle By Name(w756) -> ("ERD 3.Scaler"=w755:u32)
            n204 = Decimal String To Number(string=w754) -> (number=w757:i32)  [unwired: 2 in, 1 out]
            n205 = To Double Precision Float(number=w755) -> (double precision float=w758:dbl)
            n206 = To Double Precision Float(number=w757) -> (double precision float=w759:dbl)
            n207 = Divide(x=w759, y=w758) -> (x/y=w753:dbl)
            n208 = Bundle By Name(cluster=w746, "ERD Value 3"=w753) -> (w752:T1)
          }
          frame 50 {
            n209 = case shown="\"01\"" w768 {
              selector: w768 -> [w769 _ _]
              tunnel: [w769 "LOCKED" ("Motor Profile") "UNLOCKED" ("Motor Profile")] -> w765
              frame "0", Default {
              }
              frame "00" {
              }
              frame "01" {
              }
            }
            n210 = Bundle By Name(cluster=w767, "Lid Lock FB"=w765) -> (w766:T8)
          }
          frame 51 {
            n211 = String Subset(string=w775, offset (0)=0, length (rest)=2 ("length (rest)")) -> (substring=w793:string)
            n212 = String Subset(string=w775, offset (0)=3, length (rest)=2 ("length (rest)")) -> (substring=w792:string)
            n213 = String Subset(string=w775, offset (0)=6, length (rest)=2 ("length (rest)")) -> (substring=w780:string)
            n214 = String Subset(string=w775, offset (0)=9, length (rest)=2 ("length (rest)")) -> (substring=w781:string)
            n215 = Concatenate Strings(w793, w792) -> (w791:string)
            n216 = Concatenate Strings(w780, w781) -> (w782:string)
            n217 = Hexadecimal String To Number(string=w791) -> (number=w788:u32)  [unwired: 2 in, 1 out]
            n218 = Hexadecimal String To Number(string=w782) -> (number=w785:u32)  [unwired: 2 in, 1 out]
            n219 = To Double Precision Float(number=w788) -> (double precision float=w789:dbl)
            n220 = To Double Precision Float(number=w785) -> (double precision float=w784:dbl)
            n221 = Divide(x=w789, y=100.0) -> (x/y=w786:dbl)
            n222 = Divide(x=w784, y=100.0) -> (x/y=w774:dbl)
            n223 = Bundle By Name(cluster=w787, "Hot Gallons"=w786, "Cold Gallons"=w774) -> (w773:T3)
          }
          frame 52 {
            n224 = Decimal String To Number(string=w804) -> (number=w805:i32)  [unwired: 2 in, 1 out]
            n225 = To Double Precision Float(number=w805) -> (double precision float=w806:dbl)
            n226 = Divide(x=w806, y=10.0) -> (x/y=w803:dbl)
            n227 = Bundle By Name(cluster=w812, "Hot Inlet Temp"=w803) -> (w811:T3)
          }
          frame 53 {
            n228 = Decimal String To Number(string=w816) -> (number=w817:i32)  [unwired: 2 in, 1 out]
            n229 = To Double Precision Float(number=w817) -> (double precision float=w818:dbl)
            n230 = Divide(x=w818, y=10.0) -> (x/y=w815:dbl)
            n231 = Bundle By Name(cluster=w824, "Cold Inlet Temp"=w815) -> (w823:T3)
          }
          frame 54 {
            n232 = Decimal String To Number(string=w828) -> (number=w829:i32)  [unwired: 2 in, 1 out]
            n233 = To Double Precision Float(number=w829) -> (double precision float=w830:dbl)
            n234 = Divide(x=w830, y=10.0) -> (x/y=w827:dbl)
            n235 = Bundle By Name(cluster=w836, "Warm Inlet Temp"=w827) -> (w835:T3)
          }
          frame 55 {
            n236 = String Subset(string=w844, offset (0)=0, length (rest)=2 ("length (rest)")) -> (substring=w855:string)
            n237 = String Subset(string=w844, offset (0)=3, length (rest)=2 ("length (rest)")) -> (substring=w854:string)
            n238 = String Subset(string=w844, offset (0)=6, length (rest)=2 ("length (rest)")) -> (substring=w849:string)
            n239 = String Subset(string=w844, offset (0)=9, length (rest)=2 ("length (rest)")) -> (substring=w850:string)
            n240 = Concatenate Strings(w855, w854) -> (w853:string)
            n241 = Concatenate Strings(w849, w850) -> (w851:string)
            n242 = Hexadecimal String To Number(string=w853) -> (number=w842:u32)  [unwired: 2 in, 1 out]
            n243 = Hexadecimal String To Number(string=w851) -> (number=w840:u32)  [unwired: 2 in, 1 out]
            n244 = To Unsigned Word Integer(number=w842) -> (unsigned 16bit integer=w841:u16)
            n245 = To Unsigned Word Integer(number=w840) -> (unsigned 16bit integer=w839:u16)
            n246 = Bundle By Name(cluster=w852, "Hot Seg Valve Time"=w841, "Cold Seg Valve Time"=w839) -> (w843:T3)
          }
          frame 56 {
            n247 = Decimal String To Number(string=w865) -> (number=w866:i32)  [unwired: 2 in, 1 out]
            n248 = To Unsigned Word Integer(number=w866) -> (unsigned 16bit integer=w864:u16)
            n249 = Bundle By Name(cluster=w869, "Coast Time"=w864) -> (w868:T2)
          }
          frame 57 {
            n250 = Decimal String To Number(string=w875) -> (number=w876:i32)  [unwired: 2 in, 1 out]
            n251 = To Unsigned Word Integer(number=w876) -> (unsigned 16bit integer=w874:u16)
            n252 = Bundle By Name(cluster=w883, "Ramp Time"=w874) -> (w882:T2)
          }
          frame 58 {
            n253 = Decimal String To Number(string=w885) -> (number=w886:i32)  [unwired: 2 in, 1 out]
            n254 = To Unsigned Word Integer(number=w886) -> (unsigned 16bit integer=w884:u16)
            n255 = Bundle By Name(cluster=w893, "Ramp  Speed"=w884) -> (w892:T2)
          }
          frame 59 {
            n256 = Decimal String To Number(string=w896) -> (number=w897:i32)  [unwired: 2 in, 1 out]
            n257 = To Double Precision Float(number=w897) -> (double precision float=w898:dbl)
            n258 = Divide(x=w898, y=1024.0) -> (x/y=w895:dbl)
            n259 = Bundle By Name(cluster=w905, "Ramp Avg Current"=w895) -> (w904:T2)
          }
          frame 60 {
            n260 = Decimal String To Number(string=w907) -> (number=w908:i32)  [unwired: 2 in, 1 out]
            n261 = To Unsigned Word Integer(number=w908) -> (unsigned 16bit integer=w906:u16)
            n262 = Bundle By Name(cluster=w915, "Partial Coast Time"=w906) -> (w914:T2)
          }
          frame 61 {
            n263 = Decimal String To Number(string=w917) -> (number=w918:i32)  [unwired: 2 in, 1 out]
            n264 = To Double Precision Float(number=w918) -> (double precision float=w919:dbl)
            n265 = Divide(x=w919, y=32.0) -> (x/y=w916:dbl)
            n266 = Bundle By Name(cluster=w927, "Dry Load Size"=w916) -> (w926:T2)
          }
          frame 62 {
            n267 = Decimal String To Number(string=w929) -> (number=w930:i32)  [unwired: 2 in, 1 out]
            n268 = To Double Precision Float(number=w930) -> (double precision float=w931:dbl)
            n269 = Divide(x=w931, y=32.0) -> (x/y=w928:dbl)
            n270 = Bundle By Name(cluster=w939, "Ramp Line Voltage"=w928) -> (w938:T2)
          }
          frame 63 {
            n271 = Decimal String To Number(string=w941) -> (number=w942:i32)  [unwired: 2 in, 1 out]
            n272 = To Double Precision Float(number=w942) -> (double precision float=w943:dbl)
            n273 = Divide(x=w943, y=32.0) -> (x/y=w940:dbl)
            n274 = Bundle By Name(cluster=w951, "Coast Line Voltage"=w940) -> (w950:T2)
          }
          frame 64 {
            n275 = String Subset(string=w961, offset (0)=3, length (rest)=2 ("length (rest)")) -> (substring=w962:string)
            n276 = Hexadecimal String To Number(string=w962) -> (number=w960:u32)  [unwired: 2 in, 1 out]
            n277 = case shown="0, Default" w960 {
              tunnel: ["UNLOCKED" "LOCKED" "FAILURE"] -> w956
              frame 0, Default {
              }
              frame 1 {
              }
              frame 2 {
              }
            }
            n278 = Bundle By Name(cluster=w957, "Lid Lock Req State"=w956) -> (w955:T8)
          }
          frame 65 {
            n279 = call "HexStringToBoolean.vi"("Hex String"=w976) -> ("Boolean"=w968:bool)
            n280 = Bundle By Name(cluster=w970, "OOB Detected in Accel"=w968) -> (w969:T2)
          }
          frame 66 {
            n281 = String Subset(string=w978, offset (0)=0, length (rest)=2 ("length (rest)")) -> (substring=w988:string)
            n282 = String Subset(string=w978, offset (0)=3, length (rest)=2 ("length (rest)")) -> (substring=w987:string)
            n283 = String Subset(string=w978, offset (0)=6, length (rest)=2 ("length (rest)")) -> (substring=w980:string)
            n284 = String Subset(string=w978, offset (0)=9, length (rest)=2 ("length (rest)")) -> (substring=w979:string)
            n285 = Concatenate Strings(w988, w987, w980, w979) -> (w986:string)
            n286 = Hexadecimal String To Number(string=w986) -> (number=w985:u32)  [unwired: 2 in, 1 out]
            n287 = To Long Integer(number=w985) -> (32bit integer=w977:i32)
            n288 = Bundle By Name(cluster=w994, "Max Accel in Accel"=w977) -> (w993:T2)
          }
          frame 67 {
            n289 = String Subset(string=w1001, offset (0)=0, length (rest)=2 ("length (rest)")) -> (substring=w1011:string)
            n290 = String Subset(string=w1001, offset (0)=3, length (rest)=2 ("length (rest)")) -> (substring=w1010:string)
            n291 = String Subset(string=w1001, offset (0)=6, length (rest)=2 ("length (rest)")) -> (substring=w1003:string)
            n292 = String Subset(string=w1001, offset (0)=9, length (rest)=2 ("length (rest)")) -> (substring=w1002:string)
            n293 = Concatenate Strings(w1011, w1010, w1003, w1002) -> (w1009:string)
            n294 = Hexadecimal String To Number(string=w1009) -> (number=w1008:u32)  [unwired: 2 in, 1 out]
            n295 = To Long Integer(number=w1008) -> (32bit integer=w1000:i32)
            n296 = Bundle By Name(cluster=w1017, "Max Jerk in Accel"=w1000) -> (w1016:T2)
          }
          frame 68 {
            n297 = call "HexStringToBoolean.vi"("Hex String"=w1031) -> ("Boolean"=w1023:bool)
            n298 = Bundle By Name(cluster=w1025, "OOB Detected in S-S"=w1023) -> (w1024:T2)
          }
          frame 69 {
            n299 = String Subset(string=w1033, offset (0)=0, length (rest)=2 ("length (rest)")) -> (substring=w1043:string)
            n300 = String Subset(string=w1033, offset (0)=3, length (rest)=2 ("length (rest)")) -> (substring=w1042:string)
            n301 = String Subset(string=w1033, offset (0)=6, length (rest)=2 ("length (rest)")) -> (substring=w1035:string)
            n302 = String Subset(string=w1033, offset (0)=9, length (rest)=2 ("length (rest)")) -> (substring=w1034:string)
            n303 = Concatenate Strings(w1043, w1042, w1035, w1034) -> (w1041:string)
            n304 = Hexadecimal String To Number(string=w1041) -> (number=w1040:u32)  [unwired: 2 in, 1 out]
            n305 = To Long Integer(number=w1040) -> (32bit integer=w1032:i32)
            n306 = Bundle By Name(cluster=w1049, "Max Jerk in S-S"=w1032) -> (w1048:T2)
          }
          frame 70 {
            n307 = call "HexStringToBoolean.vi"("Hex String"=w1063) -> ("Boolean"=w1055:bool)
            n308 = Bundle By Name(cluster=w1057, "OOB Redist Req"=w1055) -> (w1056:T2)
          }
          frame 71 {
            n309 = Decimal String To Number(string=w1068) -> (number=w1069:i32)  [unwired: 2 in, 1 out]
            n310 = To Double Precision Float(number=w1069) -> (double precision float=w1070:dbl)
            n311 = Divide(x=w1070, y=1.0) -> (x/y=w1067:dbl)
            n312 = Bundle By Name(cluster=w1075, "Remaining Cycle Time (s)"=w1067) -> (w1074:T8)
          }
        }
        "Numeric" <- w69
      }
    }
  }
  "ERD_Always Show" <- w27
  "Version" <- w26
  "Redundant Micro" <- w28
  "ERD Graph  Ind" <- w32
  "ATC Data" <- w22
  "Algorithm Data 2" <- w20
  "Error Out" <- "Error In"
